vi "editDevice.vi"(8 "error in (no error)":errorcluster, 9 "S/N IN":string, 10 "Device Type In":T1=enum."k4b2", 11 "reference in":refnum<class "Project Panels.lvclass">=refnum) -> (0 "error out":errorcluster={"status"=TRUE, "code"=1556, "source"="In Place Element Structure in File Controller.lvclass:getExcelFileRefs.vi->Devices Controller.lvclass:newDevice.vi->Project Panels.lvclass:newItem.vi->Project Panels.lvclass:products.vi->GUI Controller.lvclass:operate.vi->Master Controller.lvclass:operate.vi->main.vi"}, 2 "saved?":bool, 3 "reference out":refnum<class "Project Panels.lvclass">)   [LabVIEW 2015, in "Project Panels.lvclass"]
uses:
  Project Panels.lvclass
  SYS/Devices Controller_llb/deviceType.ctl
  deviceState.ctl
  SYS/Devices Controller_llb/Devices Controller.lvclass
panel:
  out "title":string="Edit ...."
  in  "Note:":string
  in  "O2 Exp Date (mmm-yy)":string
  in  "Serviced by":string
  in  "O2 Last Changed (mmm-yy)":string
  in  "Follow Up Accepeted  (dd-mmm-yy)":string
  in  "Follow Up Sent (dd-mmm-yy)":string
  out "Device Type":T1=enum."k4b2"
  in  "City":string
  in  "End User Email":string
  in  "End User":string
  in  "System's Location":string
  in  "Account":string
  in  "Description":string
  in  "SW Version":string
  out "S/N":string
  out "statusBar":string
  in  "Save Button":bool
  in  "Stop Button":bool
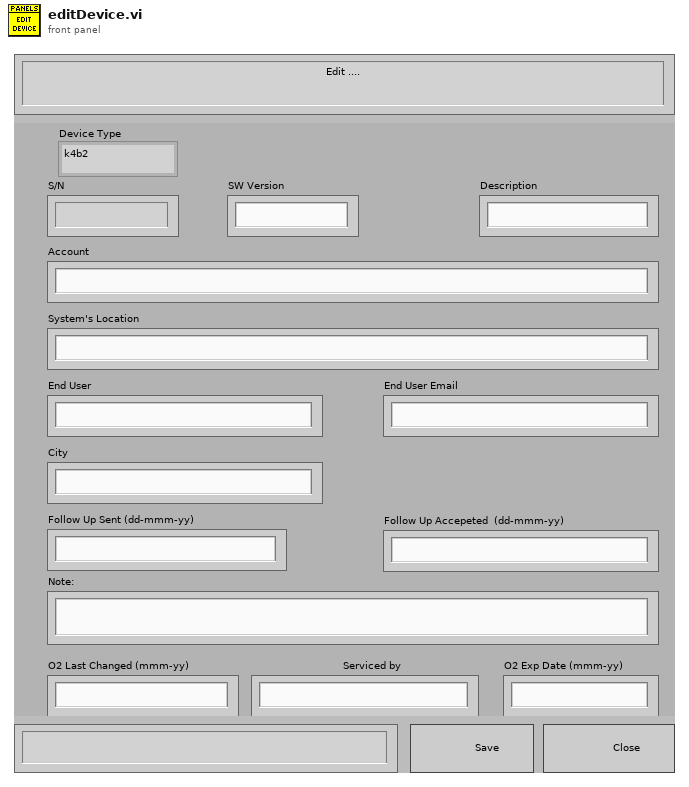
[diagram p1: front panel]
types:
  T1 = typedef "Devices Controller.lvclass/deviceType.ctl" = enum16{"k5", "k4b2", "fitmate", "cpet", "rmr", "bodyBoxPft", "bp", "pp"}
  T2 = cluster{"deviceType":T1, "S/N":string, "SW":string, "Description":string, "Account":string, "System's Location":string, "End User":string, "Email":string, "City":string, "LastChange":string, "Service By":string, "Exp Date":string, "FollowUp Sent":string, "FollowUp Accepted":string, "Note":string}
  T3 = typedef "Project Panels.lvclass/deviceState.ctl" = enum16{"check", "initiate", "waitEvent", "dataFromPDF", "getDetails", "save", "close", "stop"}
  T4 = enum8{"Enabled", "Disabled", "Disabled and Grayed Out"}
  T5 = typedef "Project Panels.lvclass/ObjectAttributesRef.ctl" = refnum<data-value>
  T6 = typedef "Project Panels.lvclass/ObjectAttributes.ctl" = cluster{"MyAttribute":dbl, "device_controller_ref":refnum<class "Devices Controller.lvclass">, "file_controller_ref":refnum<class "File Controller.lvclass">, "item_controller_ref":refnum<class "Items Controller.lvclass">, "item_tables":cluster{"checkIN":string[][], "checkOUT":string[][], "storage":string[][]}, "quickbook_table":cluster{"notes":string[][]}, "notification_controller_ref":refnum<class "Notification Controller.lvclass">, "partstracking_controller_ref":refnum<class "PartsTracking Controller.lvclass">, "product_tables":cluster{"k4b2":string[][], "fitmate":string[][], "RMR":string[][], "CPET":string[][], "BP":string[][], "PP":string[][], "k5":string[][], "bb-pft":string[][]}, "rowsColour":u32[], "low_resolution?":bool}
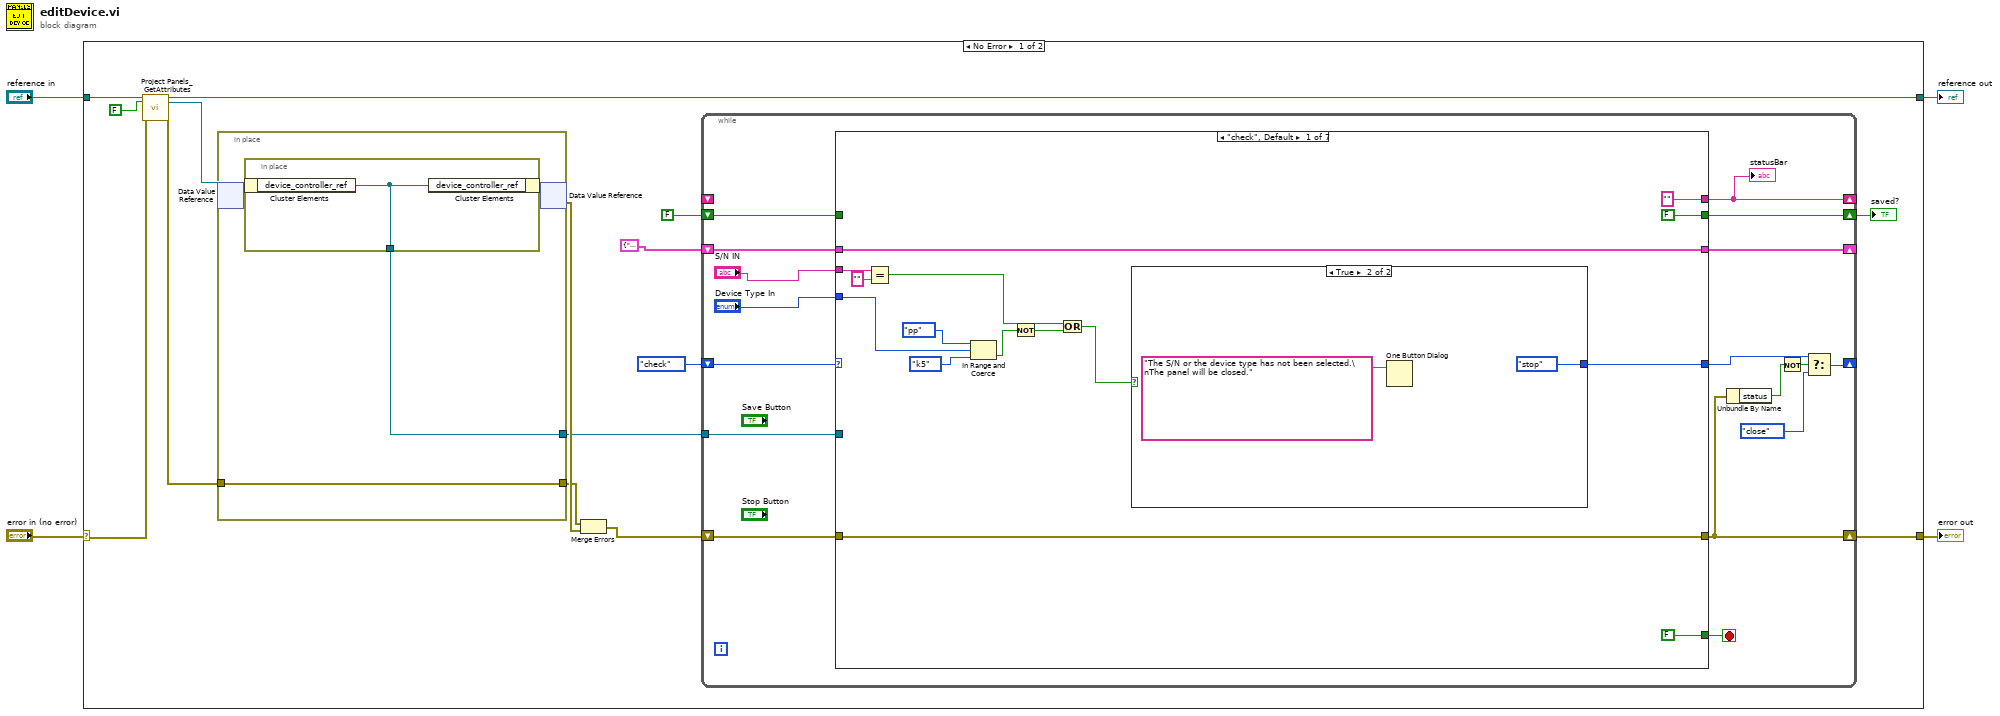
[diagram p0: block diagram]
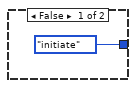
[diagram p2: hidden frame]
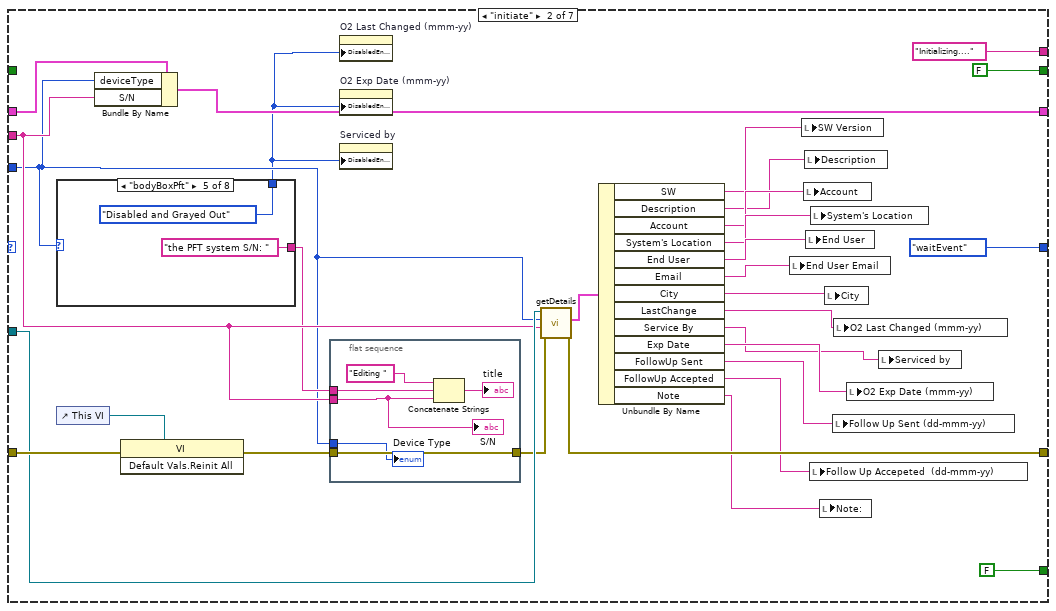
[diagram p3: hidden frame]
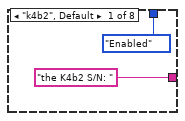
[diagram p4: hidden frame]
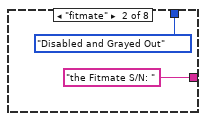
[diagram p5: hidden frame]
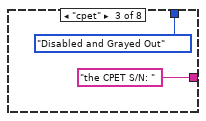
[diagram p6: hidden frame]
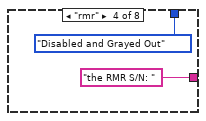
[diagram p7: hidden frame]
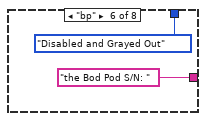
[diagram p8: hidden frame]
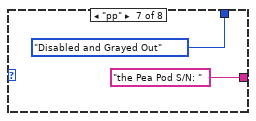
[diagram p9: hidden frame]
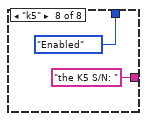
[diagram p10: hidden frame]
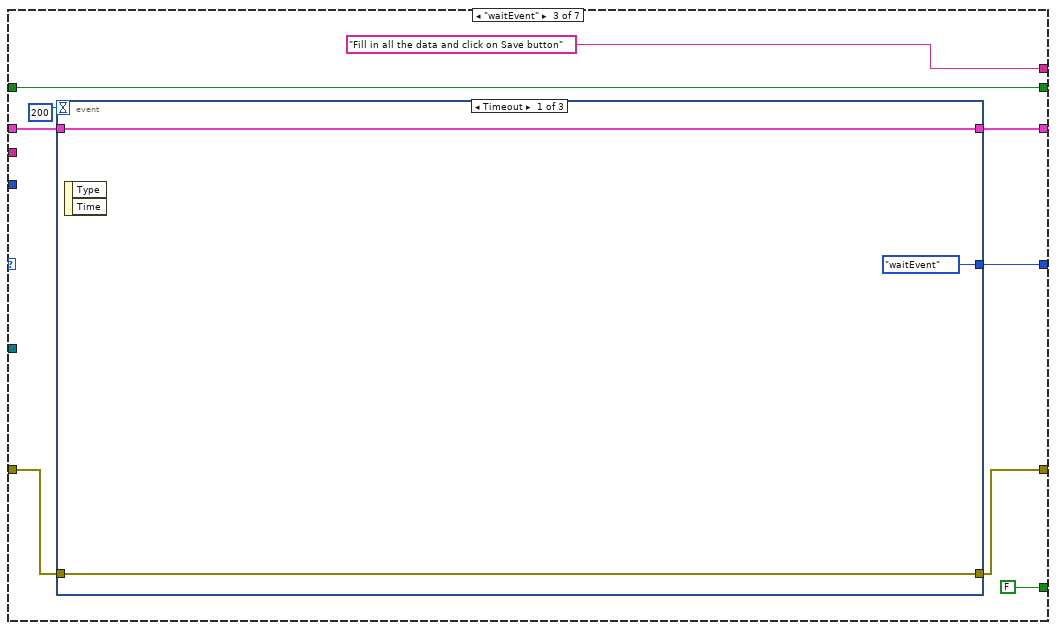
[diagram p11: hidden frame]
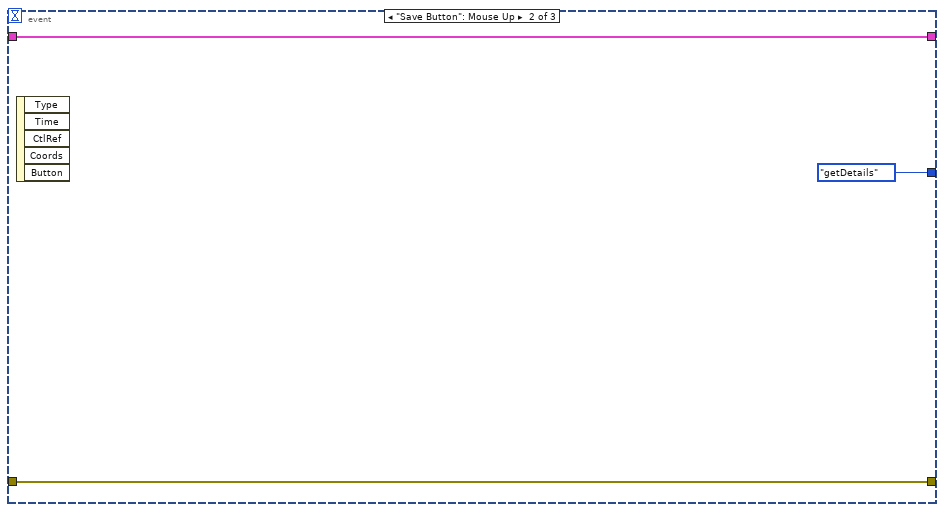
[diagram p12: hidden frame]
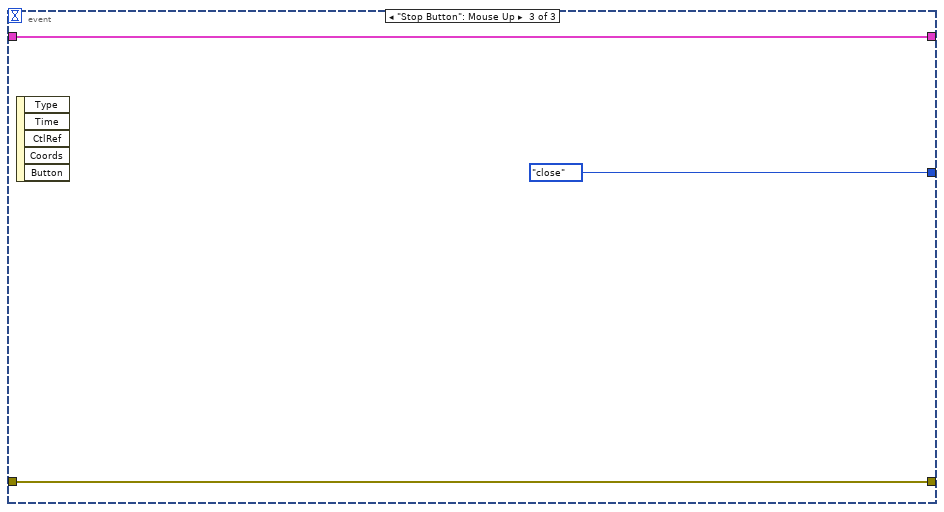
[diagram p13: hidden frame]
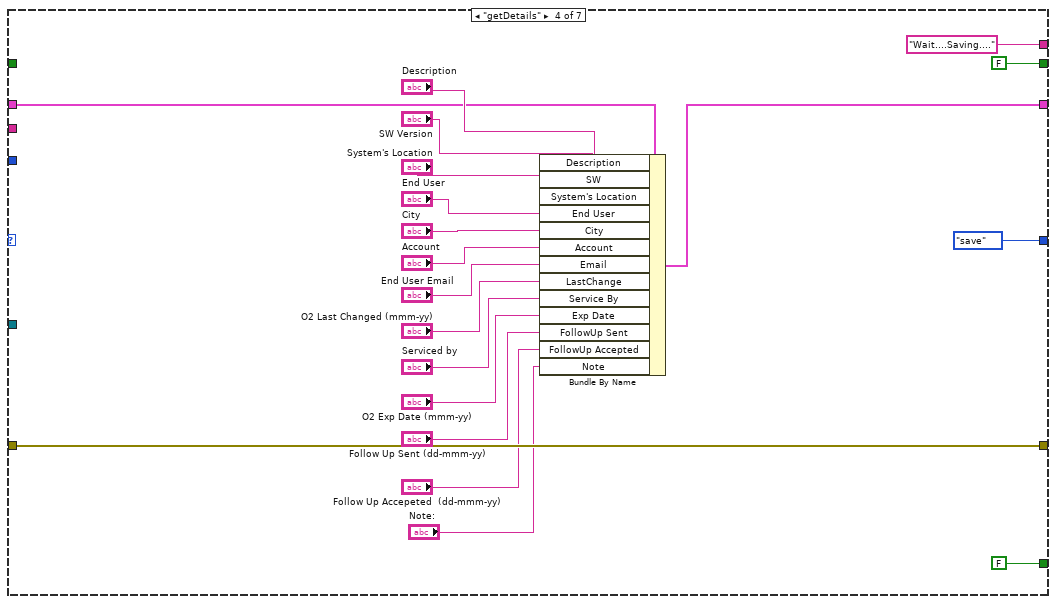
[diagram p14: hidden frame]
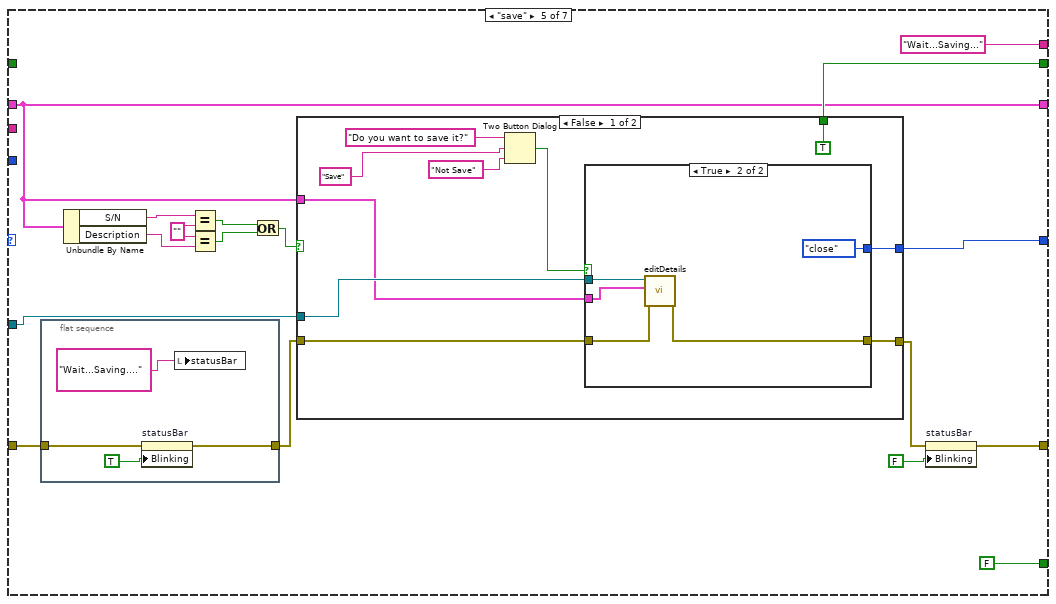
[diagram p15: hidden frame]
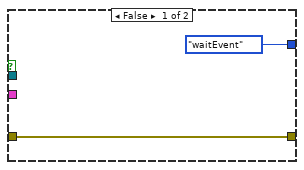
[diagram p16: hidden frame]
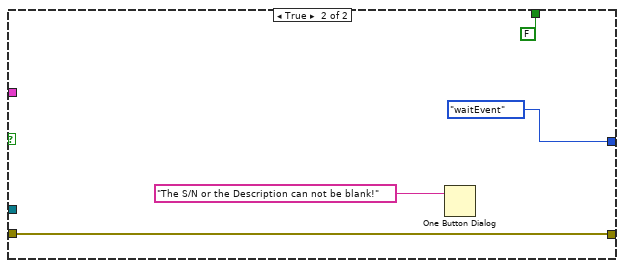
[diagram p17: hidden frame]
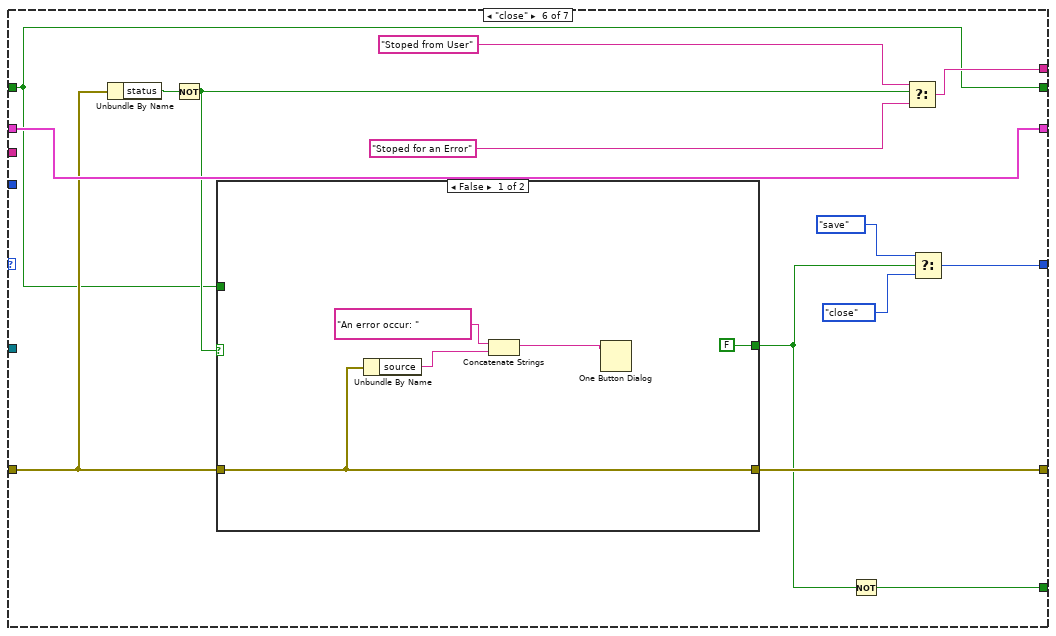
[diagram p18: hidden frame]
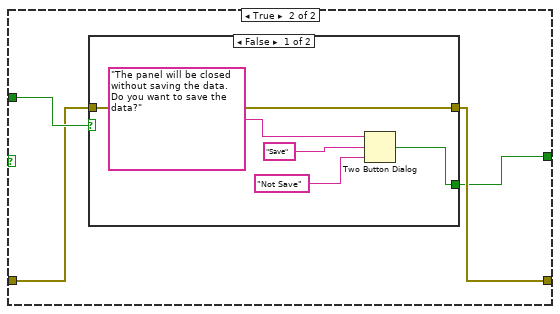
[diagram p19: hidden frame]
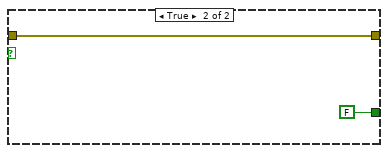
[diagram p20: hidden frame]
diagram:
  n1 = case shown="No Error" "error in (no error)" {
    selector: "error in (no error)" -> [w15 w229]
    tunnel: [w10 w229] -> w3
    tunnel: [w13 w228] -> w1
    tunnel: "reference in" -> [w17 w228]
    frame No Error {
      n2 = call "Project Panels_GetAttributes.vi"("reference in"=w17, "return data? (T)"=FALSE, "error in (no error)"=w15) -> ("reference out"=w13:refnum<class "Project Panels.lvclass">, "attributes ref"=w12:T5, "error out"=w14:errorcluster)  [unwired: 13 in, 1 out]
      n3 = in-place {
        in-place-border: w14 -> [w224]
        in-place-border: [w224] -> w18
        in-place-border: [w223] -> w8
        n4 = in-place-dvr #1(w12) -> (w225:T6)  [unwired: 1 out]
        n5 = in-place {
          in-place-border: [w227] -> w223
          n6 = in-place-cluster #2(w225) -> ("device_controller_ref"=w227:refnum<class "Devices Controller.lvclass">)
          n7 = in-place-cluster #2("device_controller_ref"=w227) -> (w226:T6)
        }
        n8 = in-place-dvr #1(w226) -> (w19:errorcluster)  [unwired: 1 out]
      }
      n9 = Merge Errors(w18, w19) -> (w11:errorcluster)
      n10 = while {
        shift-right: [w25] -> w10
        shift-left: w11 -> [w36]
        shift-right: [w26] -> _
        shift-left: deviceState."check" ("state") -> [w35]
        shift-right: [w33] -> _
        shift-left: T2 {"deviceType"=enum."k5", "S/N"="", "SW"="", "Description"="", "Account"="", "System's Location"="", "End User"="", "Email"="", "City"="", "LastChange"="", "Service By"="", "Exp Date"="", "FollowUp Sent"="", "FollowUp Accepted"="", "Note"=""} ("details") -> [w32]
        shift-right: [w31] -> _
        shift-left: _ -> [_]
        tunnel: w8 -> [w30]
        shift-right: [w29] -> w6
        shift-left: FALSE -> [w28]
        stop <- w34 stop-if-true
        n11 = case shown="\"check\", Default" w35 {
          tunnel: w36 -> [w51 w79 w110 w144 w151 w195 w221]
          tunnel: [w51 w78 w109 w144 w147 w194 w221] -> w25
          tunnel: [FALSE FALSE FALSE FALSE FALSE w189 TRUE] -> w34
          tunnel: [w39 deviceState."waitEvent" ("state") w114 deviceState."save" ("f") w155 w193 deviceState."stop" ("f")] -> w27
          tunnel: "Device Type In" -> [w47 w57 _ _ _ _ _]
          tunnel: [w48 w62 w107 w128 w152 w197 w219] -> w33
          tunnel: w32 -> [w48 w63 w108 w129 w152 w197 w219]
          tunnel: ["" ("title") "Initializing...." ("statusBar") "Fill in all the data and click on Save button" ("statusBar") "Wait....Saving...." ("title") "Wait...Saving..." ("title") w196 "" ("title")] -> w31
          tunnel: w30 -> [_ w77 _ _ w154 _ _]
          tunnel: [FALSE FALSE w111 FALSE w153 w187 FALSE] -> w29
          tunnel: w28 -> [_ _ w111 _ _ w187 _]
          tunnel: "S/N IN" -> [w45 w61 _ _ _ _ _]
          frame "check", Default {
            n12 = Equal?(x=w45, y="") -> (x = y?=w42:bool)
            n13 = In Range and Coerce(upper limit=deviceType."pp", x=w47, lower limit=deviceType."k5") -> (In Range?=w43:bool)  [unwired: 1 out]
            n14 = Not(x=w43) -> (.not. x?=w41:bool)
            n15 = Or(x=w42, y=w41) -> (x .or. y?=w40:bool)
            n16 = case shown="True" w40 {
              tunnel: [deviceState."initiate" ("f") deviceState."stop" ("f")] -> w39
              frame False {
              }
              frame True {
                n17 = One Button Dialog(message="The S/N or the device type has not been selected.\nThe panel will be closed.") -> ()  [unwired: 1 in, 1 out]
              }
            }
          }
          frame "initiate" {
            n18 = case shown="\"bodyBoxPft\"" w57 {
              tunnel: ["the K4b2 S/N: " ("string") "the Fitmate S/N: " ("string") "the CPET S/N: " ("string") "the RMR S/N: " ("string") "the PFT system S/N: " ("string") "the Bod Pod S/N: " ("string") "the Pea Pod S/N: " ("string") "the K5 S/N: " ("string")] -> w60
              tunnel: [T4."Enabled" ("Disabled") T4."Disabled and Grayed Out" ("Disabled") T4."Disabled and Grayed Out" ("Disabled") T4."Disabled and Grayed Out" ("Disabled") T4."Disabled and Grayed Out" ("Disabled") T4."Disabled and Grayed Out" ("Disabled") T4."Disabled and Grayed Out" ("Disabled") T4."Enabled" ("Disabled")] -> w55
              frame "k4b2", Default {
              }
              frame "fitmate" {
              }
              frame "cpet" {
              }
              frame "rmr" {
              }
              frame "bodyBoxPft" {
              }
              frame "bp" {
              }
              frame "pp" {
              }
              frame "k5" {
              }
            }
            n19 = control-ref of="This VI"() -> (w80:refnum<vi>)
            n20 = Bundle By Name(cluster=w63, "deviceType"=w57, "S/N"=w61) -> (w62:T2)
            n21 = invoke class="VI" method="Default Vals.Reinit All"(reference=w80, error in=w79) -> (error out=w59:errorcluster)  [unwired: 1 in, 2 out]
            n22 = flat-sequence {
              tunnel: w61 -> [w86]
              tunnel: w60 -> [w88]
              tunnel: w59 -> [w87]
              tunnel: [w87] -> w58
              tunnel: w57 -> [w85]
              frame #0 {
                n23 = Concatenate Strings("Editing " ("title"), w88, w86) -> (→"title":string)
                "S/N" <- w86
                "Device Type" <- w85
              }
            }
            n24 = property on="O2 Last Changed (mmm-yy)" class="Str"("DisabledEnum"=w55) -> ()  [unwired: 2 in, 2 out]
            n25 = property on="O2 Exp Date (mmm-yy)" class="Str"("DisabledEnum"=w55) -> ()  [unwired: 2 in, 2 out]
            n26 = property on="Serviced by" class="Str"("DisabledEnum"=w55) -> ()  [unwired: 2 in, 2 out]
            n27 = call "getDetails.vi"("error in (no error)"=w58, "S/N"=w61, "Device Type"=w57, "reference in"=w77) -> ("error out"=w78:errorcluster, "details"=w76:T2)  [unwired: 5 in, 1 out]
            n28 = Unbundle By Name(w76) -> ("SW"=w70:string, "Description"=w71:string, "Account"=w72:string, "System's Location"=w73:string, "End User"=w74:string, "Email"=w75:string, "City"=w69:string, "LastChange"=w68:string, "Service By"=w64:string, "Exp Date"=w65:string, "FollowUp Sent"=w66:string, "FollowUp Accepted"=w67:string, "Note"=w56:string)
            n29 = local write "End User Email"(w75) -> ()
            n30 = local write "SW Version"(w70) -> ()
            n31 = local write "Account"(w72) -> ()
            n32 = local write "Description"(w71) -> ()
            n33 = local write "End User"(w74) -> ()
            n34 = local write "Follow Up Accepeted  (dd-mmm-yy)"(w67) -> ()
            n35 = local write "System's Location"(w73) -> ()
            n36 = local write "Note:"(w56) -> ()
            n37 = local write "City"(w69) -> ()
            n38 = local write "Follow Up Sent (dd-mmm-yy)"(w66) -> ()
            n39 = local write "O2 Last Changed (mmm-yy)"(w68) -> ()
            n40 = local write "O2 Exp Date (mmm-yy)"(w65) -> ()
            n41 = local write "Serviced by"(w64) -> ()
          }
          frame "waitEvent" {
            n42 = event shown="[0] Timeout" {
              selector: _ -> [_ _ _]
              dyn-events: _ -> [_ _ _]
              timeout: 200 -> [_ _ _]
              tunnel: [deviceState."waitEvent" ("state") deviceState."getDetails" ("state") deviceState."close" ("state")] -> w114
              tunnel: [w117 w120 w123] -> w109
              tunnel: w110 -> [w117 w120 w123]
              tunnel: w108 -> [w116 w119 w122]
              tunnel: [w116 w119 w122] -> w107
              event Timeout {
                n43 = event-data() -> ()  [unwired: 1 in, 2 out]
              }
              event "Save Button": Mouse Up {
                n44 = event-data() -> ()  [unwired: 1 in, 5 out]
              }
              event "Stop Button": Mouse Up {
                n45 = event-data() -> ()  [unwired: 1 in, 5 out]
              }
            }
          }
          frame "getDetails" {
            n46 = Bundle By Name(cluster=w129, "Description"="Description", "SW"="SW Version", "System's Location"="System's Location", "End User"="End User", "City"="City", "Account"="Account", "Email"="End User Email", "LastChange"="O2 Last Changed (mmm-yy)", "Service By"="Serviced by", "Exp Date"="O2 Exp Date (mmm-yy)", "FollowUp Sent"="Follow Up Sent (dd-mmm-yy)", "FollowUp Accepted"="Follow Up Accepeted  (dd-mmm-yy)", "Note"="Note:") -> (w128:T2)
          }
          frame "save" {
            w159 = "" ("y")
            n47 = flat-sequence {
              tunnel: [w163] -> w150
              tunnel: w151 -> [w164]
              frame #0 {
                n48 = property on="statusBar" class="Str"(error in=w164, "Blinking"=TRUE) -> (error out=w163:errorcluster)  [unwired: 1 in, 1 out]
                n49 = local write "statusBar"("Wait...Saving...." ("statusBar")) -> ()
              }
            }
            n50 = Unbundle By Name(w152) -> ("S/N"=w148:string, "Description"=w160:string)
            n51 = Equal?(x=w148, y=w159) -> (x = y?=w158:bool)
            n52 = Equal?(x=w159, y=w160) -> (x = y?=w157:bool)
            n53 = Or(x=w158, y=w157) -> (x .or. y?=w156:bool)
            n54 = case shown="False" w156 {
              tunnel: w150 -> [w173 w183]
              tunnel: [w170 w183] -> w146
              tunnel: [w175 deviceState."waitEvent" ("state")] -> w155
              tunnel: w154 -> [w172 _]
              tunnel: [TRUE FALSE] -> w153
              tunnel: w152 -> [w171 _]
              frame False {
                n55 = Two Button Dialog(message="Do you want to save it?", 1:"Not Save" ("F button name (\"Cancel\")"), 2:"Save" ("T button name (\"OK\")")) -> (T button?=w168:bool)
                n56 = case shown="True" w168 {
                  tunnel: [deviceState."waitEvent" ("state") deviceState."close" ("state")] -> w175
                  tunnel: w173 -> [w177 w181]
                  tunnel: w172 -> [_ w180]
                  tunnel: w171 -> [_ w179]
                  tunnel: [w177 w178] -> w170
                  frame False {
                  }
                  frame True {
                    n57 = call "editDetails.vi"("error in (no error)"=w181, "details"=w179, "reference in"=w180) -> ("error out"=w178:errorcluster)  [unwired: 7 in, 1 out]
                  }
                }
              }
              frame True {
                n58 = One Button Dialog(message="The S/N or the Description can not be blank!") -> ()  [unwired: 1 in, 1 out]
              }
            }
            n59 = property on="statusBar" class="Str"(error in=w146, "Blinking"=FALSE) -> (error out=w147:errorcluster)  [unwired: 1 in, 1 out]
          }
          frame "close" {
            n60 = Unbundle By Name(w195) -> ("status"=w200:bool)
            n61 = Not(x=w200) -> (.not. x?=w188:bool)
            n62 = case shown="False" w188 {
              tunnel: w187 -> [_ w209]
              tunnel: w195 -> [w202 w208]
              tunnel: [w202 w207] -> w194
              tunnel: [FALSE ("Save") w206] -> w190
              frame False {
                n63 = Unbundle By Name(w202) -> ("source"=w201:string)
                n64 = Concatenate Strings("An error occur: " ("message"), w201) -> (w203:string)
                n65 = One Button Dialog(message=w203) -> ()  [unwired: 1 in, 1 out]
              }
              frame True {
                n66 = case shown="False" w209 {
                  tunnel: w208 -> [w214 w215]
                  tunnel: [w214 w215] -> w207
                  tunnel: [w212 FALSE ("Save")] -> w206
                  frame False {
                    n67 = Two Button Dialog(message="The panel will be closed without saving the data. Do you want to save the data?", 1:"Not Save" ("F button name (\"Cancel\")"), 2:"Save" ("T button name (\"OK\")")) -> (T button?=w212:bool)
                  }
                  frame True {
                  }
                }
              }
            }
            n68 = Not(x=w190) -> (.not. x?=w189:bool)
            n69 = Select(t="Stoped from User" ("title"), s=w188, f="Stoped for an Error" ("title")) -> (s? t:f=w196:string)
            n70 = Select(t=deviceState."save" ("state"), s=w190, f=deviceState."close" ("state")) -> (s? t:f=w193:T3)
          }
          frame "stop" {
          }
        }
        "statusBar" <- w31
        n71 = Unbundle By Name(w25) -> ("status"=w24:bool)
        n72 = Not(x=w24) -> (.not. x?=w22:bool)
        n73 = Select(t=w27, s=w22, f=deviceState."close") -> (s? t:f=w26:T3)
      }
      "saved?" <- w6
    }
    frame Error {
    }
  }
  "error out" <- w3
  "reference out" <- w1
